vi "transfer_and_submit_job.vi"(7 "Date Folder":string, 8 "Password":string, 9 "Username":string, 10 "Remote Data Directory":string, 11 "Local Data Directory":string) -> ()   [LabVIEW 2014]
panel:
  out "standard error":string
  out "standard output":string
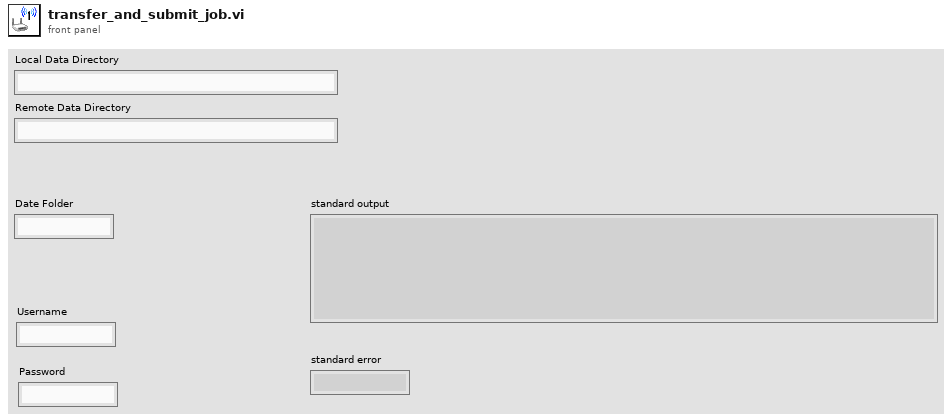
[diagram p1: front panel]
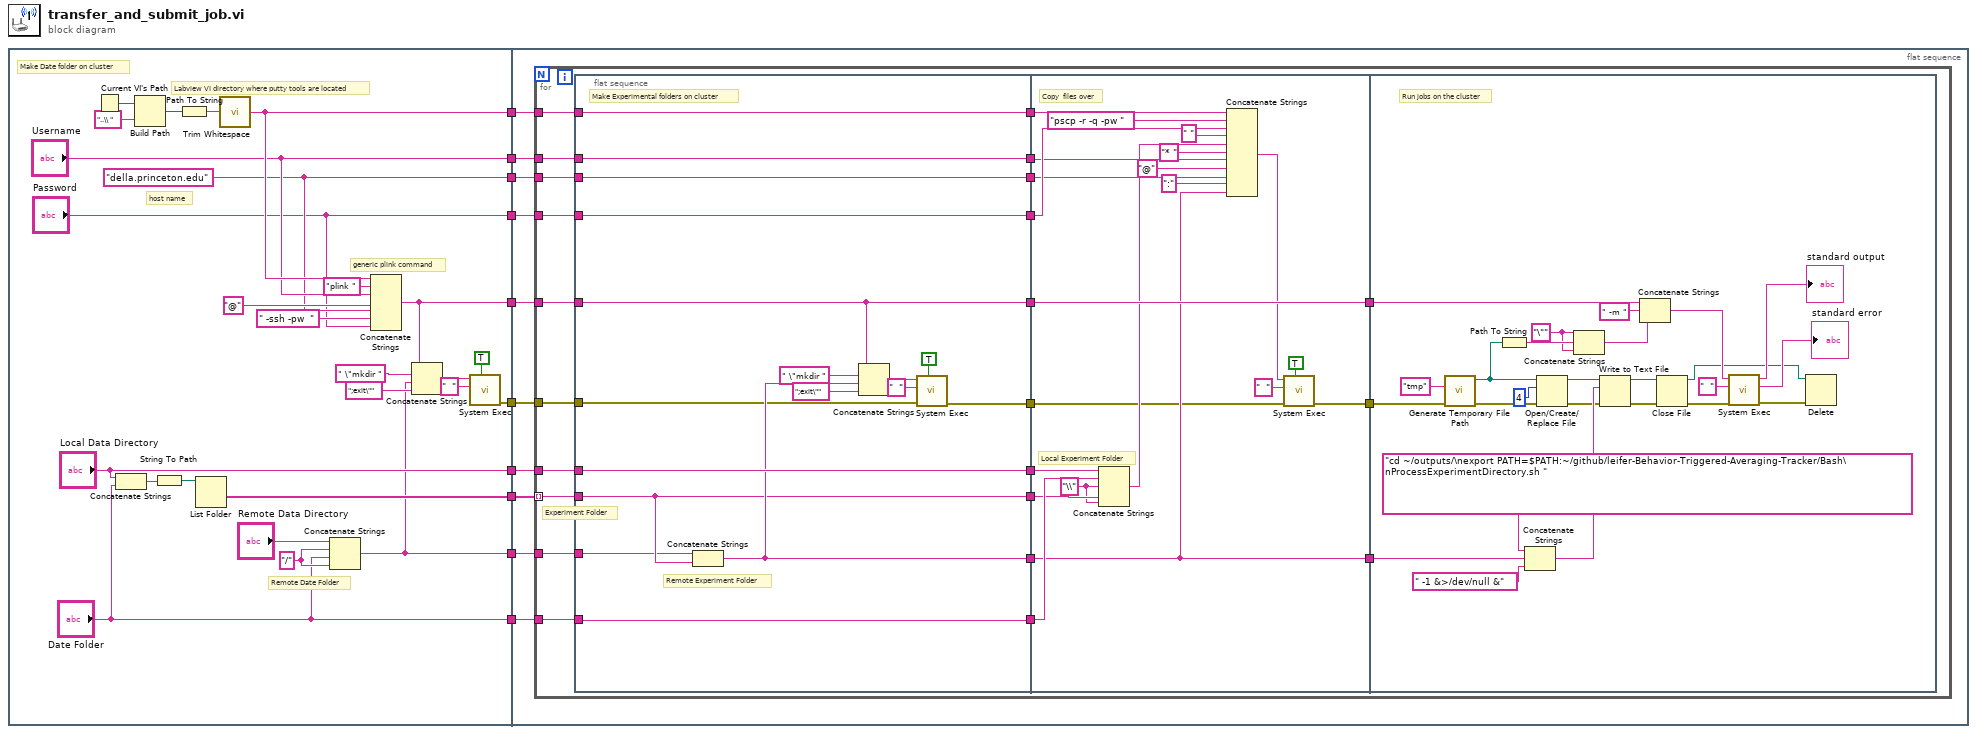
[diagram p0: block diagram]
diagram:
  n1 = flat-sequence {
    tunnel: ["Local Data Directory"] -> w10
    tunnel: [w33] -> w9
    tunnel: [w20] -> w8
    tunnel: ["Username"] -> w7
    tunnel: [w18] -> w6
    tunnel: ["Password"] -> w5
    tunnel: [w16] -> w4
    tunnel: ["Date Folder"] -> w3
    tunnel: [w12] -> w2
    tunnel: [w11] -> w1
    tunnel: w10 -> [w40]
    tunnel: w9 -> [w39]
    tunnel: w8 -> [w46]
    tunnel: w7 -> [w45]
    tunnel: w6 -> [w44]
    tunnel: w5 -> [w43]
    tunnel: w4 -> [w42]
    tunnel: w3 -> [w37]
    tunnel: w2 -> [w38]
    tunnel: w1 -> [w41]
    frame #0 {
      w14 = "/"
      w18 = "della.princeton.edu"
      # "generic plink command"
      # "host name"
      # "Make Date folder on cluster"
      # "Remote Date Folder"
      # "Labview VI directory where putty tools are located"
      n2 = Current VI's Path() -> (path=w29:path)
      n3 = Concatenate Strings("Local Data Directory", "Date Folder") -> (w35:string)
      n4 = Build Path(base path=w29, name or relative path="..\\ ") -> (appended path=w31:path)
      n5 = String To Path(string=w35) -> (path=w34:path)
      n6 = Path To String(path=w31) -> (string=w32:string)
      n7 = List Folder(path=w34) -> (folder names=w33:string[])  [unwired: 3 in, 3 out]
      n8 = call <vilib>:"Trim Whitespace.vi"("string"=w32) -> ("trimmed string"=w20:string)  [unwired: 1 in]
      n9 = Concatenate Strings("Remote Data Directory", w14, "Date Folder", w14) -> (w12:string)
      n10 = Concatenate Strings(w20, "plink ", "Username", "@", w18, " -ssh -pw  ", "Password") -> (w16:string)
      n11 = Concatenate Strings(w16, " \"mkdir ", w12, ";exit\"") -> (w21:string)
      n12 = call <vilib>:"System Exec.vi"("wait until completion? (T)"=TRUE, "standard input"="  ", "command line"=w21) -> ("error out"=w11:errorcluster)  [unwired: 5 in, 3 out]
    }
    frame #1 {
      n13 = for {
        tunnel: w37 -> [w69]
        tunnel: w40 -> [w68]
        tunnel: w39 -> [w67] mode=indexing
        tunnel: w46 -> [w60]
        tunnel: w45 -> [w52]
        tunnel: w44 -> [w51]
        tunnel: w43 -> [w50]
        tunnel: w42 -> [w49]
        tunnel: w38 -> [w48]
        tunnel: w41 -> [w47]
        # "Experiment Folder"
        n14 = flat-sequence {
          tunnel: [w76] -> w65
          tunnel: w69 -> [w76]
          tunnel: w67 -> [w77]
          tunnel: [w77] -> w66
          tunnel: w68 -> [w84]
          tunnel: [w75] -> w64
          tunnel: [w73] -> w63
          tunnel: [w74] -> w62
          tunnel: [w85] -> w61
          tunnel: w60 -> [w85]
          tunnel: [w84] -> w59
          tunnel: [w81] -> w57
          tunnel: [w72] -> w55
          tunnel: [w78] -> w54
          tunnel: w52 -> [w75]
          tunnel: w51 -> [w74]
          tunnel: w50 -> [w73]
          tunnel: w49 -> [w72]
          tunnel: w48 -> [w71]
          tunnel: w47 -> [w70]
          tunnel: w66 -> [w100]
          tunnel: w65 -> [w106]
          tunnel: w64 -> [w95]
          tunnel: w63 -> [w102]
          tunnel: w62 -> [w94]
          tunnel: w61 -> [w103]
          tunnel: w59 -> [w107]
          tunnel: [w92] -> w58
          tunnel: w57 -> [w92]
          tunnel: [w105] -> w56
          tunnel: w55 -> [w105]
          tunnel: w54 -> [w88]
          tunnel: [w87] -> w53
          tunnel: w58 -> [w112]
          tunnel: w56 -> [w111]
          tunnel: w53 -> [w110]
          frame #0 {
            # "Remote Experiment Folder"
            # "Make Experimental folders on cluster"
            n15 = Concatenate Strings(w71, w77) -> (w81:string)
            n16 = Concatenate Strings(w72, " \"mkdir ", w81, ";exit\"") -> (w79:string)
            n17 = call <vilib>:"System Exec.vi"("wait until completion? (T)"=TRUE, "error in (no error)"=w70, "standard input"="  ", "command line"=w79) -> ("error out"=w78:errorcluster)  [unwired: 4 in, 3 out]
          }
          frame #1 {
            w99 = "\\"
            # "Local Experiment Folder"
            # "Copy  files over"
            n18 = Concatenate Strings(w107, w106, w99, w100, w99) -> (w98:string)
            n19 = Concatenate Strings(w103, "pscp -r -q -pw ", w102, " ", w98, "* ", w95, "@", w94, ":", w92) -> (w89:string)
            n20 = call <vilib>:"System Exec.vi"("wait until completion? (T)"=TRUE, "error in (no error)"=w88, "standard input"="  ", "command line"=w89) -> ("error out"=w87:errorcluster)  [unwired: 4 in, 3 out]
          }
          frame #2 {
            w108 = "\""
            # "Run jobs on the cluster"
            n21 = call <vilib>:"Generate Temporary File Path.vi"("error in (no error)"=w110, "Temporary File Extension (tmp)"="tmp") -> ("error out"=w118:errorcluster, "Unique Temporary File Path"=w124:path)  [unwired: 8 in]
            n22 = Path To String(path=w124) -> (string=w109:string)
            n23 = Concatenate Strings("cd ~/outputs/\nexport PATH=$PATH:~/github/leifer-Behavior-Triggered-Averaging-Tracker/Bash\nProcessExperimentDirectory.sh ", w112, " -1 &>/dev/null &") -> (w126:string)
            n24 = Open/Create/Replace File(file path (use dialog)=w124, error in=w118, operation (0:open)=4) -> (refnum out=w119:refnum<file>, error out=w116:errorcluster)  [unwired: 3 in, 1 out]
            n25 = Concatenate Strings(w108, w109, w108) -> (w115:string)
            n26 = Write to Text File(file (use dialog)=w119, text=w126, error in=w116) -> (refnum out=w120:refnum<file>, error out=w117:errorcluster)  [unwired: 1 in, 1 out]
            n27 = Concatenate Strings(w111, " -m ", w115) -> (w127:string)
            n28 = Close File(refnum=w120, error in=w117) -> (error out=w121:errorcluster)  [unwired: 1 out]
            n29 = call <vilib>:"System Exec.vi"("error in (no error)"=w121, "standard input"="  ", "command line"=w127) -> ("error out"=w122:errorcluster, "standard error"=→"standard error":string, "standard output"=→"standard output":string)  [unwired: 5 in, 1 out]
            n30 = Delete(path (use dialog)=w124, error in=w122) -> ()  [unwired: 3 in, 3 out]
          }
        }
      }
    }
  }
